vi "StopSync.vi"(8 "error in (no error)":errorcluster, 11 "PXI_MultiTrig in":refnum<class "PXI_MultiTrig.lvclass">) -> (0 "error out":errorcluster, 3 "PXI_MultiTrig out":refnum<class "PXI_MultiTrig.lvclass">)   [LabVIEW 2018, in "SyncPlugins.lvlib" / "PXI_MultiTrig.lvclass"]
uses:
  PXI_MultiTrig.lvclass
  <vilib>/nisyscfg/nisyscfg.lvlib
  <vilib>/nisyscfg/Close (System).vi
  <vilib>/nisyscfg/Close (Hardware).vi
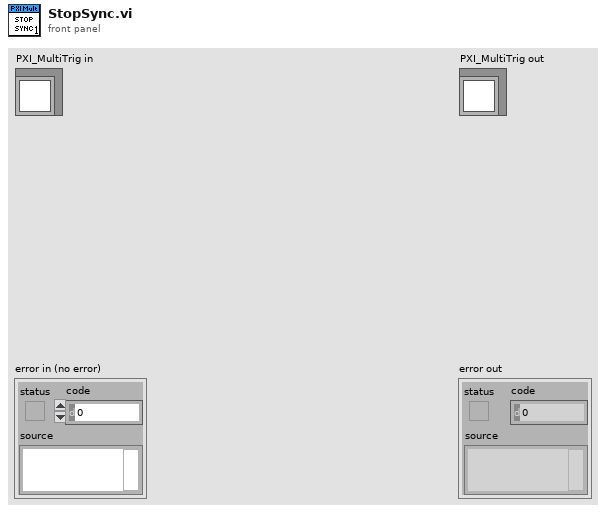
[diagram p1: front panel]
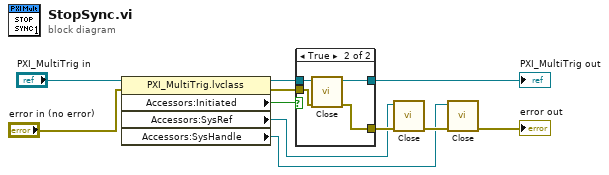
[diagram p0: block diagram]
diagram:
  n1 = property class="PXI_MultiTrig.lvclass"(reference="PXI_MultiTrig in", error in="error in (no error)") -> (reference out=w9:refnum<class "PXI_MultiTrig.lvclass">, error out=w7:errorcluster, "Accessors:Initiated"=w6:bool, "Accessors:SysRef"=w3:refnum<k20>, "Accessors:SysHandle"=w2:refnum<k21>)
  n2 = case shown="True" w6 {
    tunnel: [w13 w17] -> w11
    tunnel: [w12 w16] -> w5
    tunnel: w9 -> [w13 w15]
    tunnel: w7 -> [w12 w14]
    frame False {
    }
    frame True {
      n3 = call-dynamic <vilib>:"Close.vi"("error in (no error)"=w14, "PXI_MultiTrig in"=w15) -> ("error out"=w16:errorcluster, "PXI_MultiTrig out"=w17:refnum<class "PXI_MultiTrig.lvclass">)  [unwired: 8 in]
    }
  }
  "PXI_MultiTrig out" <- w11
  n4 = call-poly <vilib>:"Close.vi"("error in (no error)"=w5, "Resource in"=w3) -> ("error out"=w4:errorcluster)  [unwired: 9 in]
  n5 = call-poly <vilib>:"Close.vi"("error in (no error)"=w4, "Session in"=w2) -> ("error out"=→"error out":errorcluster)  [unwired: 9 in]
